vi "Problem1.10-ExecutionTime.vi"() -> ()   [LabVIEW 2019]
uses:
  <vilib>/Analysis/baseanly.llb/Mean (DBL).vi
  <vilib>/Analysis/NI_AALBase.lvlib
panel:
  out "Execution Time (ms)":dbl
  out "Random Number Array":dbl[](array[numeric])
  out "Histogram":dynamicdata(graph)
  out "Uniform Deviate Array":dbl[](array[numeric])
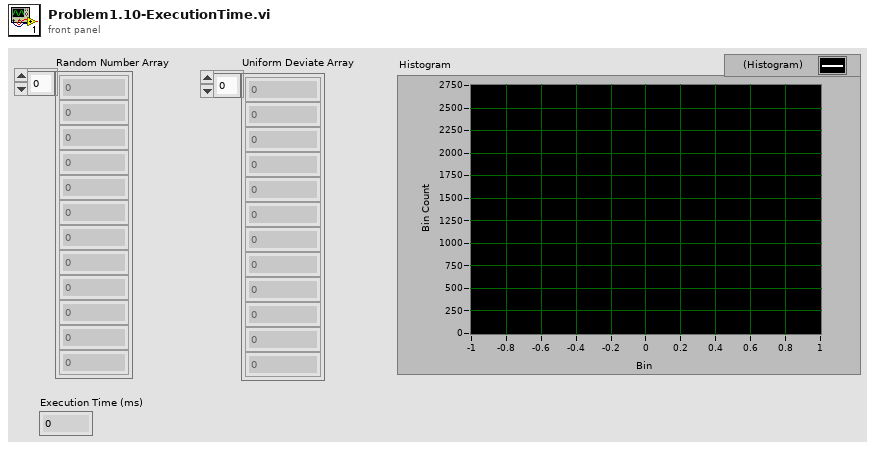
[diagram p1: front panel]
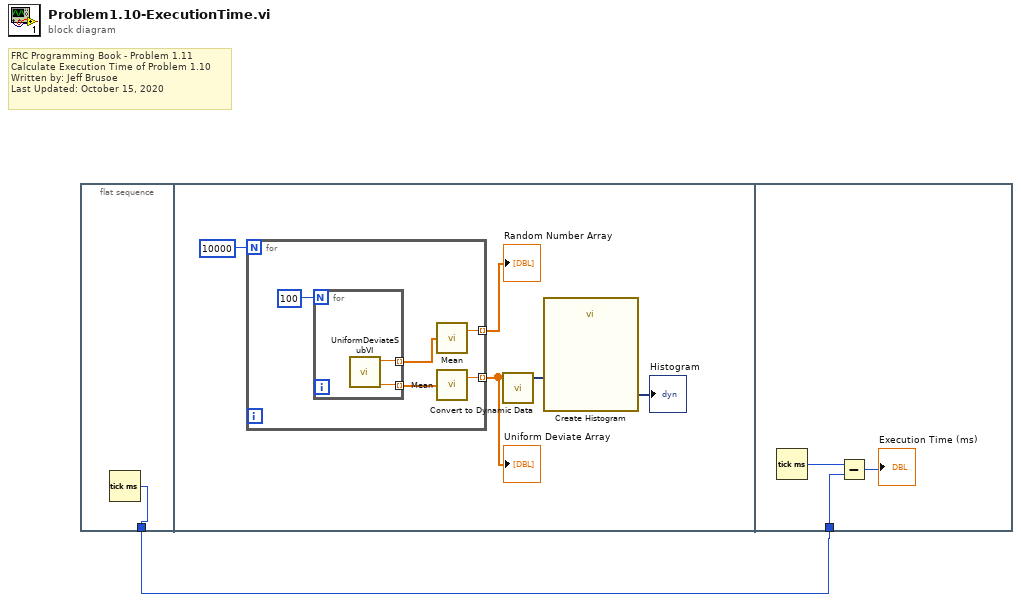
[diagram p0: block diagram]
diagram:
  # "FRC Programming Book - Problem 1.11\nCalculate Execution Time of Problem 1.10\nWritten by: Jeff Brusoe\nLast Updated: October 15, 2020"
  n1 = flat-sequence {
    tunnel: [w2] -> w1
    tunnel: w1 -> [w15]
    frame #0 {
      n2 = Tick Count (ms)() -> (millisecond timer value=w2:u32)
    }
    frame #1 {
      n3 = for {
        N: 10000 -> [_]
        tunnel: [w10] -> w4 mode=indexing
        tunnel: [w8] -> w3 mode=indexing
        n4 = for {
          N: 100 -> [_]
          tunnel: [w13] -> w11 mode=indexing
          tunnel: [w14] -> w9 mode=indexing
          n5 = call "UniformDeviateSubVI.vi"() -> ("Uniform Deviate"=w13:dbl, "Initial Random Number"=w14:dbl)  [unwired: 10 in]
        }
        n6 = call-poly <vilib>:"Mean.vi"("X"=w9) -> ("mean"=w8:dbl)  [unwired: 1 out]
        n7 = call-poly <vilib>:"Mean.vi"("X"=w11) -> ("mean"=w10:dbl)  [unwired: 1 out]
      }
      "Uniform Deviate Array" <- w4
      "Random Number Array" <- w3
      n8 = call "Convert to Dynamic Data"("Array"=w4) -> ("Dynamic Data Type"=w6:dynamicdata)  [unwired: 3 in]
      n9 = call "Create Histogram"("Signal"=w6) -> ("Histogram"=→"Histogram":dynamicdata)  [unwired: 9 in, 1 out]
    }
    frame #2 {
      n10 = Tick Count (ms)() -> (millisecond timer value=w16:u32)
      n11 = Subtract(x=w16, y=w15) -> (x-y=→"Execution Time (ms)":u32)
    }
  }
